vi "[GV]_오브젝트화된 물체 수.vi"() -> ()   [LabVIEW 2016, in "Lidar Variables.lvlib"]
uses:
  Lidar Variables.lvlib
panel:
  in  "오브젝트화된 물체 수":i16
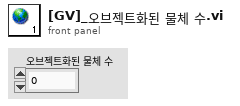
[diagram p1: front panel]
diagram:
